vi "start_subsystem_pv.vi"(6 "configuration":T1={"enable_mrc"=0, "hologram_composition"=1, "recording_indicator"=0, "video_stabilization"=0, "blank_protected"=0, "show_mesh"=0, "shared"=0, "_reserved_0"=0, "global_opacity"=0.9, "output_width"=0.0, "output_height"=0.0, "video_stabilization_length"=0, "hologram_perspective"=1, "_reserved_1"=0}, 9 "port":u16, 10 "host":string, 11 "path in":path=path "hl2ss_ulm.dll") -> (0 "error":bool, 1 "port":u16, 2 "host":string, 3 "path out":path, 4 "configuration":T1)   [LabVIEW 2023]
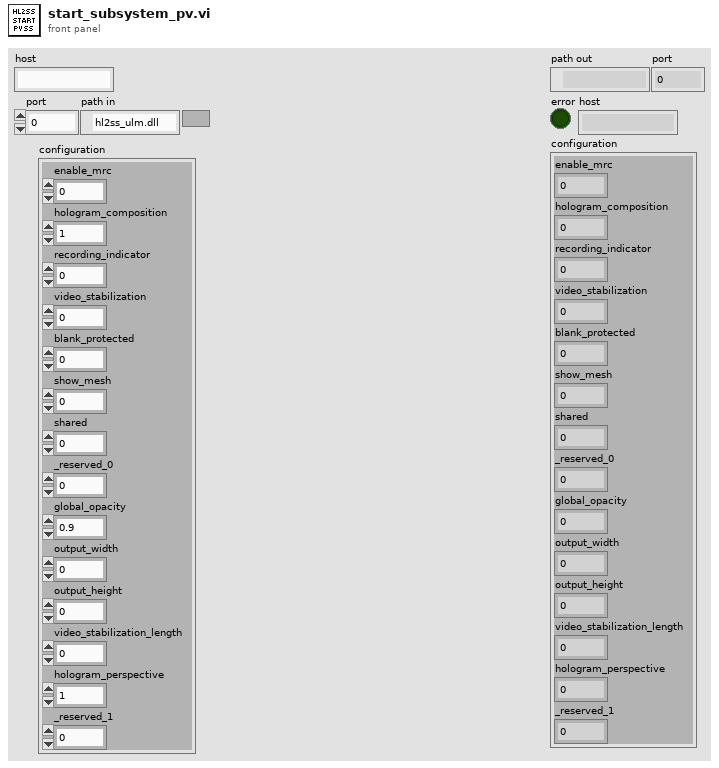
[diagram p1: front panel]
types:
  T1 = cluster{"enable_mrc":u8, "hologram_composition":u8, "recording_indicator":u8, "video_stabilization":u8, "blank_protected":u8, "show_mesh":u8, "shared":u8, "_reserved_0":u8, "global_opacity":sgl, "output_width":sgl, "output_height":sgl, "video_stabilization_length":u32, "hologram_perspective":u32, "_reserved_1":u32}
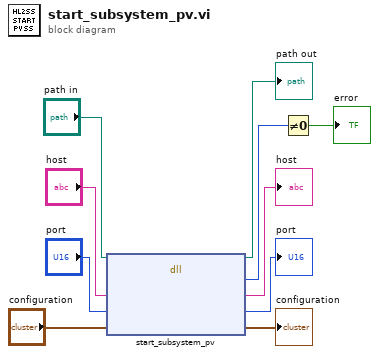
[diagram p0: block diagram]
diagram:
  n1 = dll-call lib="C:/Users/jcds/Documents/GitHub/hl2ss/extensions/client_labview/hl2ss_ulm.dll" fn="start_subsystem_pv"(path in="path in", "host"="host", "port"="port", "configuration"="configuration") -> (path out=→"path out":path, "return type"=w6:i32, "host"=→"host":string, "port"=→"port":u16, "configuration"=→"configuration":T1)  [unwired: 2 in, 1 out]
  n2 = Not Equal To 0?(x=w6) -> (x != 0?=→"error":bool)
